vi "Initialize Calibration.vi"(8 "error in (no error)":errorcluster, 10 "SignalCluster":T1, 11 "Queue in":refnum<queue>) -> (0 "error out":errorcluster, 2 "SignalCluster out":T1, 3 "Queue out":refnum<queue>)   [LabVIEW 2013, in "main.lvlib"]
uses:
  main.lvlib
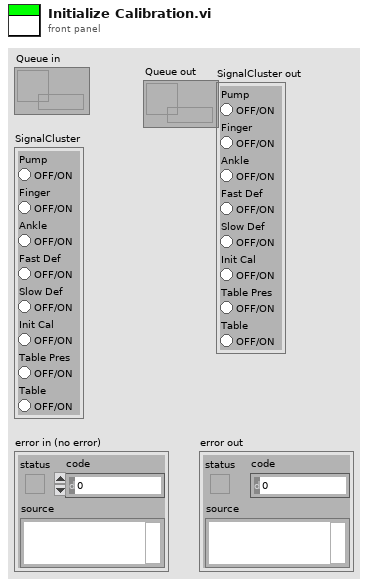
[diagram p1: front panel]
types:
  T1 = cluster{"Pump":bool, "Finger":bool, "Ankle":bool, "Fast Def":bool, "Slow Def":bool, "Init Cal":bool, "Table Pres":bool, "Table":bool}
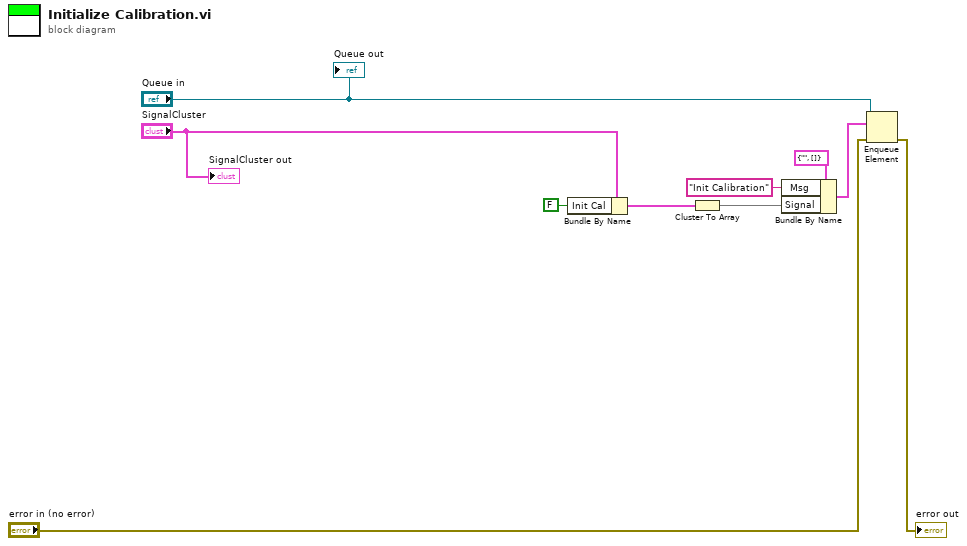
[diagram p0: block diagram]
diagram:
  n1 = Bundle By Name(cluster="SignalCluster", "Init Cal"=FALSE ("Fast Def")) -> (w9:T1)
  n2 = Cluster To Array(cluster=w9) -> (array=w8:bool[])
  n3 = Bundle By Name(cluster=cluster{"Msg":string, "Signal":bool[]} {"Msg"="", "Signal"=[]} ("element"), "Msg"="Init Calibration", "Signal"=w8) -> (w5:cluster{"Msg":string, "Signal":bool[]})
  n4 = Enqueue Element(queue="Queue in", element=w5, error in (no error)="error in (no error)") -> (error out=→"error out":errorcluster)  [unwired: 1 in, 2 out]
  "Queue out" <- "Queue in"
  "SignalCluster out" <- "SignalCluster"
